vi "onGetVarietal.vi"(8 "error in (no error)":errorcluster, 11 "Leaf.Properties in":refnum<class "Leaf.Properties.lvclass">) -> (0 "error out":errorcluster, 2 "Varietal":string, 3 "Leaf.Properties out":refnum<class "Leaf.Properties.lvclass">)   [LabVIEW 2021, in "Banana.Caraya.lvlib" / "Leaf.Properties.lvclass"]
uses:
  Leaf.Properties.lvclass
  C:/Program Files (x86)/National Instruments/LabVIEW 2021/vi.lib/addons/_JKI Toolkits/Caraya/classes/Properties/Properties.lvclass
  <vilib>/addons/_JKI Toolkits/Caraya/classes/Properties/Properties.lvclass/Properties.ctl
  <vilib>/LabVIEW Open Source Project/Cryptographic Functions/SHA-1/SHA-1.vi
  <vilib>/LabVIEW Open Source Project/Cryptographic Functions/SHA-1/SHA-1.lvclass
  <vilib>/LabVIEW Open Source Project/Cryptographic Functions/SHA-1/SHA-1.lvlib
  <vilib>/addons/_JKI Toolkits/Caraya/classes/Properties/Properties.lvclass
  <vilib>/addons/_JKI Toolkits/Caraya/classes/Basic Test Manager/Basic Test Manager.lvclass
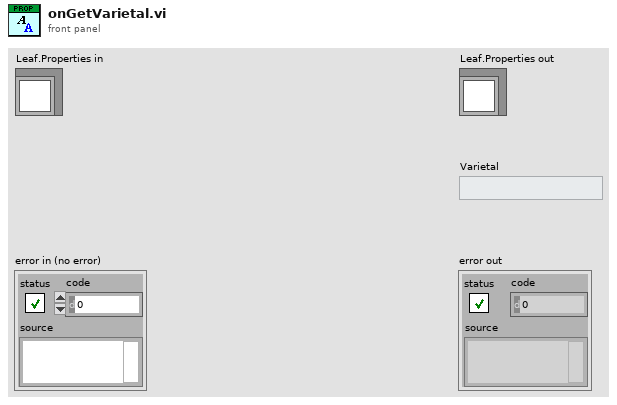
[diagram p1: front panel]
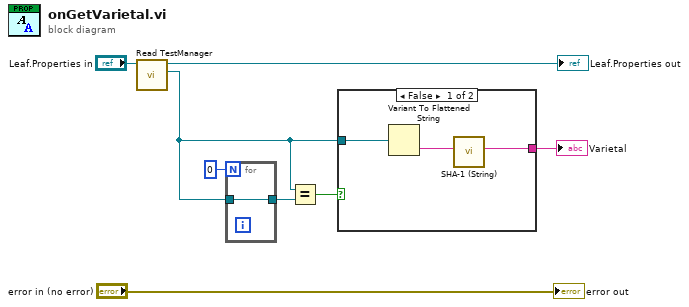
[diagram p0: block diagram]
diagram:
  n1 = call <vilib>:"Read TestManager.vi"("Properties in"="Leaf.Properties in") -> ("Test Manager"=w1:refnum<class "Basic Test Manager.lvclass">, "Properties out"=→"Leaf.Properties out":refnum<class "Leaf.Properties.lvclass">)  [unwired: 9 in]
  n2 = for {
    N: 0 -> [_]
    tunnel: [w9] -> w6
    tunnel: w1 -> [w9]
  }
  n3 = Equal?(x=w1, y=w6) -> (x = y?=w7:bool)
  n4 = case shown="False" w7 {
    tunnel: [w12 _] -> w4
    tunnel: w1 -> [w10 _]
    frame False {
      n5 = Variant To Flattened String(Variant=w10) -> (data string=w11:string)  [unwired: 1 out]
      n6 = call <vilib>:"SHA-1 (String).vi"("message"=w11) -> ("SHA-1 hash"=w12:string)  [unwired: 10 in]
    }
    frame True {
    }
  }
  "Varietal" <- w4
  "error out" <- "error in (no error)"
